vi "affichage d'un signal aleatoire (Xx10)+L.vi"() -> ()   [LabVIEW 2014]
panel:
  in  "stop":bool
  out "Waveform Chart":dbl(graph)
  in  "periode s":dbl(knob) scale=0.0..10.0
  in  "Button Rotatif":dbl(knob) scale=0.0..100.0
  # "affichage d'un signal aléatoire"
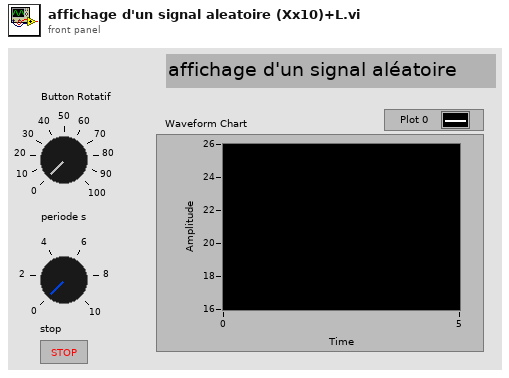
[diagram p1: front panel]
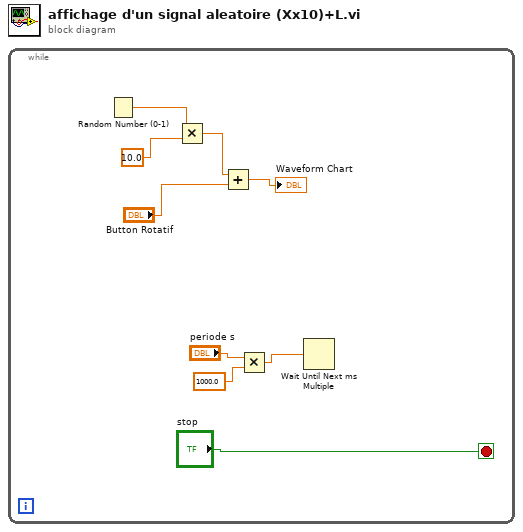
[diagram p0: block diagram]
diagram:
  n1 = while {
    stop <- "stop" stop-if-true
    n2 = Random Number (0-1)() -> (number: 0 to 1=w9:dbl)
    n3 = Multiply(x=w9, y=10.0) -> (x*y=w7:dbl)
    n4 = Add(x=w7, y="Button Rotatif") -> (x+y=→"Waveform Chart":dbl)
    n5 = Multiply(x="periode s", y=1000.0) -> (x*y=w3:dbl)
    n6 = Wait Until Next ms Multiple(millisecond multiple=w3) -> ()  [unwired: 1 out]
  }
